vi "Add Dependencies to TargetItem.vi"(7 "Add to Project":bool=TRUE caption="Add to Project (T)", 8 "error in (no error)":errorcluster, 11 "Builder in":refnum<class "Builder.lvclass">) -> (0 "error out":errorcluster, 3 "Builder out":refnum<class "Builder.lvclass">)   [LabVIEW 2019, in "Builder.lvclass"]
uses:
  Builder/Builder.lvclass
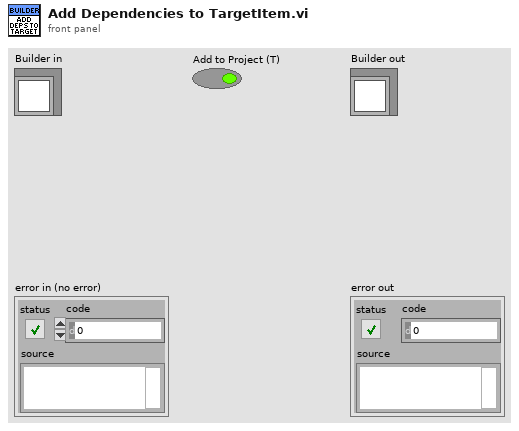
[diagram p1: front panel]
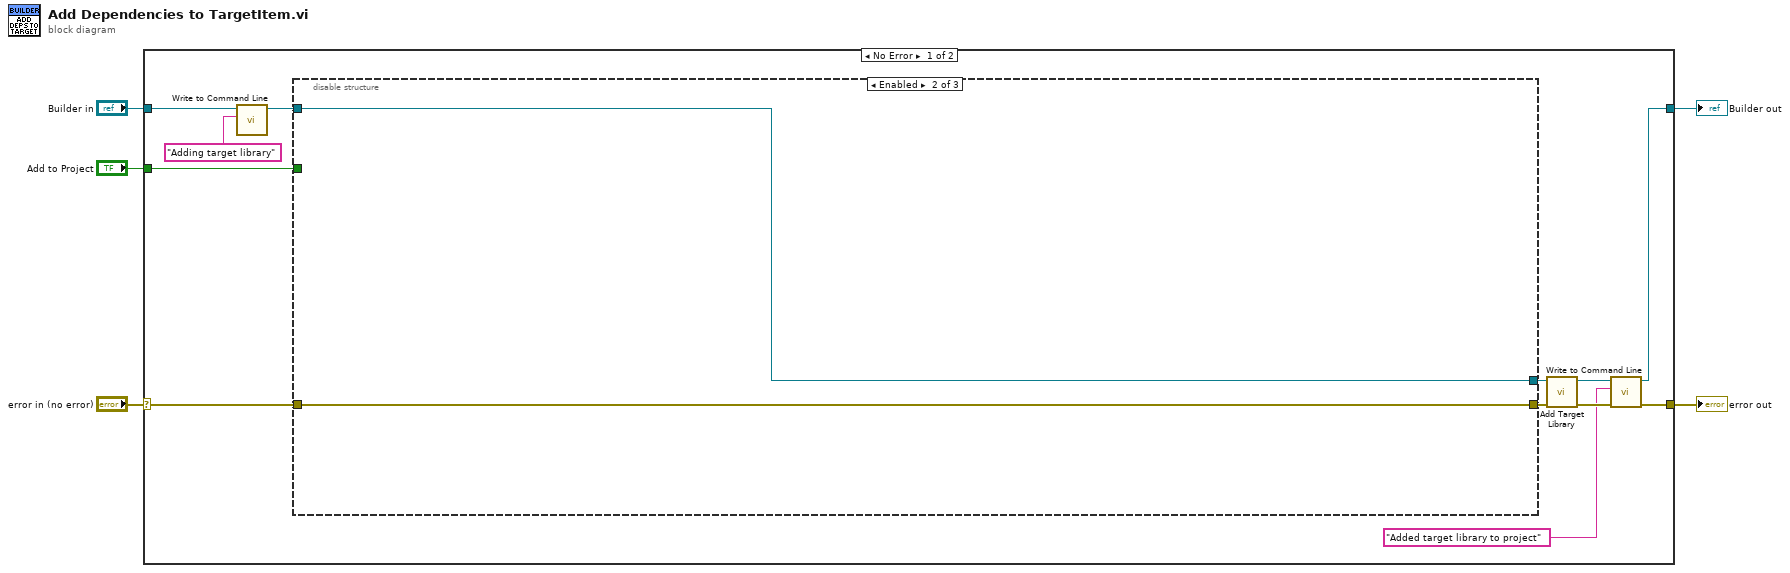
[diagram p0: block diagram]
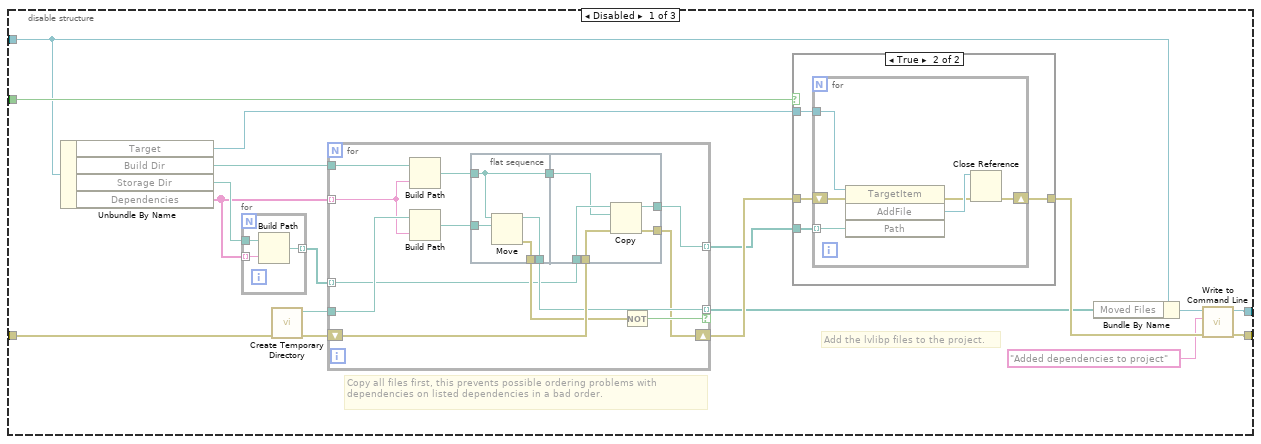
[diagram p2: hidden frame]
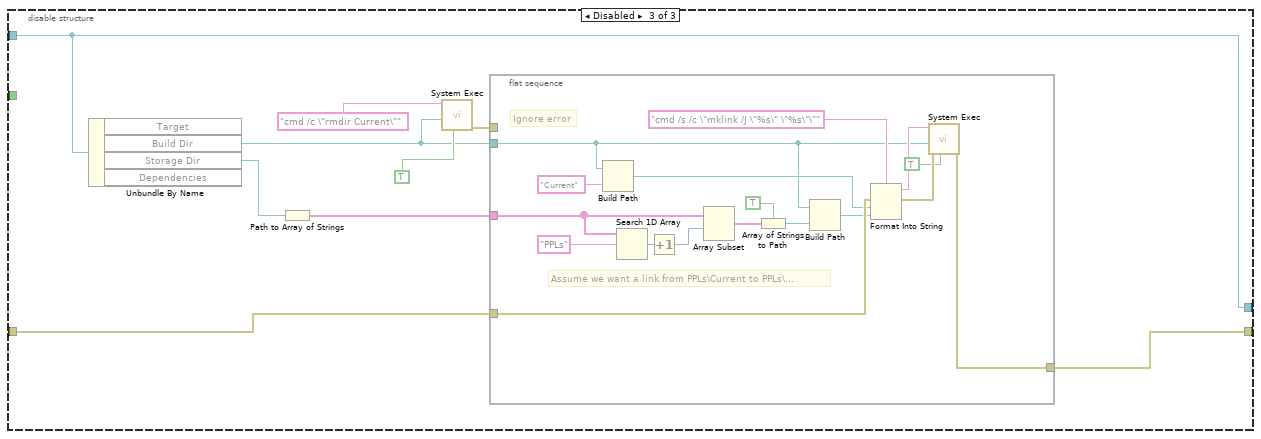
[diagram p4: hidden frame]
diagram:
  n1 = case shown="No Error" "error in (no error)" {
    selector: "error in (no error)" -> [w15 w101]
    tunnel: [w11 w101] -> w5
    tunnel: "Add to Project" -> [w16 _]
    tunnel: [w9 w100] -> w3
    tunnel: "Builder in" -> [w17 w100]
    frame No Error {
      n2 = call "Write to Command Line.vi"("Message"="Adding target library", "Builder in"=w17) -> ("Builder out"=w7:refnum<class "Builder.lvclass">)  [unwired: 8 in, 1 out]
      n3 = disable-structure shown="Enabled" {
        disable-tunnel: w7 -> [w22 w73 w76]
        disable-tunnel: w16 -> [w30 _ _]
        disable-tunnel: w15 -> [w27 w72 w80]
        disable-tunnel: [w24 w73 w76] -> w14
        disable-tunnel: [w23 w72 w81] -> w13
        frame Disabled {
          # "Add the lvlibp files to the project."
          # "Copy all files first, this prevents possible ordering problems with dependencies on listed dependencies in a bad order."
          n4 = Unbundle By Name(w22) -> ("Target"=w21:refnum<vi>, "Build Dir"=w20:path, "Storage Dir"=w19:path, "Dependencies"=w18:string[])
          n5 = for {
            tunnel: w18 -> [w38] mode=indexing
            tunnel: w19 -> [w37]
            tunnel: [w36] -> w29 mode=indexing
            n6 = Build Path(base path=w37, name or relative path=w38) -> (appended path=w36:path)
          }
          n7 = call "Create Temporary Directory.vi"("error in"=w27) -> ("error out"=w34:errorcluster, "created path"=w35:path)  [unwired: 9 in]
          n8 = for {
            tunnel: w29 -> [w50] mode=indexing
            tunnel: w20 -> [w62]
            tunnel: w35 -> [w61]
            tunnel: [w56] -> w28 mode=indexing if=w54
            tunnel: [w52] -> w32 mode=indexing
            tunnel: w18 -> [w51] mode=indexing
            shift-right: [w53] -> w33
            shift-left: w34 -> [w59]
            n9 = Build Path(base path=w62, name or relative path=w51) -> (appended path=w58:path)
            n10 = Build Path(base path=w61, name or relative path=w51) -> (appended path=w60:path)
            n11 = flat-sequence {
              tunnel: w58 -> [w65]
              tunnel: w60 -> [w66]
              tunnel: [w65] -> w57
              tunnel: [w64] -> w56
              tunnel: [w63] -> w55
              tunnel: w59 -> [w71]
              tunnel: w50 -> [w70]
              tunnel: w57 -> [w69]
              tunnel: [w68] -> w53
              tunnel: [w67] -> w52
              frame #0 {
                n12 = Move(source path=w65, 10:w66) -> (error out=w63:errorcluster, 3:w64:path)  [unwired: 3 in, 1 out]
              }
              frame #1 {
                n13 = Copy(8:w71, 10:w69, 11:w70) -> (0:w68:errorcluster, 3:w67:path)  [unwired: 2 in, 1 out]
              }
            }
            n14 = Not(x=w55) -> (.not. x?=w54:bool)
          }
          n15 = case shown="True" w30 {
            tunnel: w21 -> [_ w40]
            tunnel: w33 -> [w39 w43]
            tunnel: w32 -> [_ w42]
            tunnel: [w39 w41] -> w31
            frame False {
            }
            frame True {
              n16 = for {
                tunnel: w42 -> [w48] mode=indexing
                shift-right: [w47] -> w41
                shift-left: w43 -> [w49]
                tunnel: w40 -> [w44]
                n17 = invoke class="TargetItem" method="AddFile"(reference=w44, error in=w49, "Path"=w48) -> (error out=w45:errorcluster, "AddFile"=w46:refnum<vi>)  [unwired: 1 in, 2 out]
                n18 = Close Reference(reference=w46, error in (no error)=w45) -> (error out=w47:errorcluster)
              }
            }
          }
          n19 = Bundle By Name(cluster=w22, "Moved Files"=w28) -> (w26:refnum<class "Builder.lvclass">)
          n20 = call "Write to Command Line.vi"("error in (no error)"=w31, "Message"="Added dependencies to project" ("Text to Write"), "Builder in"=w26) -> ("error out"=w23:errorcluster, "Builder out"=w24:refnum<class "Builder.lvclass">)  [unwired: 7 in]
        }
        frame Enabled {
        }
        frame Disabled {
          n21 = Unbundle By Name(w76) -> ("Build Dir"=w75:path, "Storage Dir"=w74:path)  [unwired: 2 out]
          n22 = Path to Array of Strings(0:w74) -> (2:w82:string[])  [unwired: 1 out]
          n23 = call <vilib>:"System Exec.vi"("run minimized? (F)"=TRUE, "working directory"=w75, "command line"="cmd /c \"rmdir Current\"") -> ("error out"=w77:errorcluster)  [unwired: 5 in, 3 out]
          n24 = flat-sequence {
            tunnel: w82 -> [w98]
            tunnel: [w92] -> w81
            tunnel: w80 -> [w90]
            tunnel: w75 -> [w85]
            tunnel: w77 -> [_]
            frame #0 {
              # "Ignore error"
              # "Assume we want a link from PPLs\\Current to PPLs\\..."
              n25 = Build Path(base path=w85, name or relative path="Current") -> (appended path=w86:path)
              n26 = Search 1D Array(1D array=w98, element="PPLs") -> (index of element=w97:i32)  [unwired: 1 in]
              n27 = Increment(x=w97) -> (x+1=w88:i32)
              n28 = Array Subset(array=w98, index=w88) -> (w95:string[])  [unwired: 1 in]
              n29 = Array of Strings to Path(0:w95, 1:TRUE ("relative")) -> (2:w84:path)
              n30 = Build Path(base path=w85, name or relative path=w84) -> (appended path=w83:path)
              n31 = Format Into String(format string="cmd /s /c \"mklink /J \"%s\" \"%s\"\"" ("command line"), error in=w90, w86, w83) -> (resulting string=w93:string, error out=w91:errorcluster)  [unwired: 1 in]
              n32 = call <vilib>:"System Exec.vi"("run minimized? (F)"=TRUE, "error in (no error)"=w91, "working directory"=w85, "command line"=w93) -> ("error out"=w92:errorcluster)  [unwired: 4 in, 3 out]
            }
          }
        }
      }
      n33 = call "Add Target Library.vi"("error in (no error)"=w13, "Builder in"=w14) -> ("error out"=w12:errorcluster, "Builder out"=w10:refnum<class "Builder.lvclass">)  [unwired: 8 in]
      n34 = call "Write to Command Line.vi"("error in (no error)"=w12, "Message"="Added target library to project", "Builder in"=w10) -> ("error out"=w11:errorcluster, "Builder out"=w9:refnum<class "Builder.lvclass">)  [unwired: 7 in]
    }
    frame Error {
    }
  }
  "error out" <- w5
  "Builder out" <- w3
